vi "Destroy Py Object.vi"(8 "error in (no error)":errorcluster, 10 "Python Object Refnum":T1, 11 "Session Handle in":refnum<data-value>) -> (0 "error out":errorcluster, 3 "Session Handle out":refnum<data-value>)   [LabVIEW 2020, in "G-Embedded-Python-Interpreter-Toolkit.lvlib"]
uses:
  G-Embedded-Python-Interpreter-Toolkit.lvlib
  Python Object Reference.ctl
  Python Object Type.ctl
  bin/gepit.cp310.32.dll
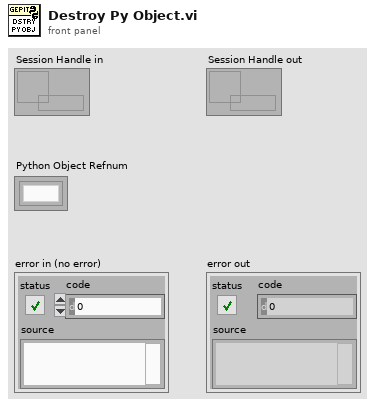
[diagram p1: front panel]
types:
  T1 = typedef "G-Embedded-Python-Interpreter-Toolkit.lvlib/Python Object Reference.ctl" = refnum<k1>
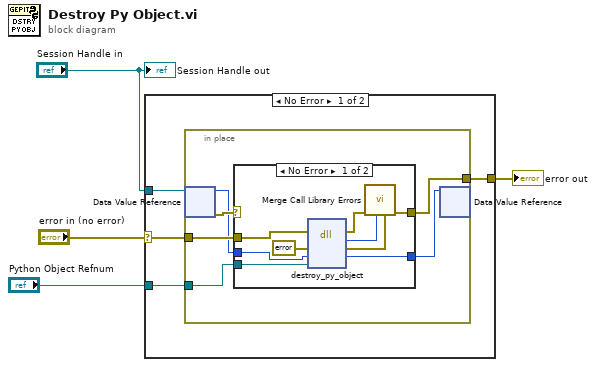
[diagram p0: block diagram]
diagram:
  n1 = case shown="No Error" "error in (no error)" {
    selector: "error in (no error)" -> [w7 w26]
    tunnel: "Session Handle in" -> [w8 _]
    tunnel: [w6 w26] -> w3
    tunnel: "Python Object Refnum" -> [w5 _]
    frame No Error {
      n2 = in-place {
        in-place-border: w7 -> [w13]
        in-place-border: [w10] -> w6
        in-place-border: w5 -> [w9]
        n3 = in-place-dvr #1(w8) -> (w12:u64, w14:errorcluster)
        n4 = case shown="No Error" w14 {
          selector: w14 -> [_ w24]
          tunnel: w13 -> [w19 _]
          tunnel: w12 -> [w18 w25]
          tunnel: [w17 w25] -> w11
          tunnel: [w16 w24] -> w10
          tunnel: w9 -> [w15 _]
          frame No Error {
            n5 = dll-call lib="C:/serenial/libraries/g-embedded-python-interpreter-toolkit/LabVIEW/bin/gepit.cp310.32.dll" fn="destroy_py_object"(error in=w19, "Error"=errorcluster {"status"=FALSE, "code"=0, "source"=""} ("error constant"), "Session"=w18, "Py Object"=w15) -> (error out=w22:errorcluster, "return type"=w21:i32, "Error"=w20:errorcluster, "Session"=w17:u64)  [unwired: 3 in, 1 out]
            n6 = call "Merge Call Library Errors.vi"("Call Library Error"=w20, "Return Value"=w21, "error in"=w22) -> ("error out"=w16:errorcluster)  [unwired: 8 in]
          }
          frame Error {
          }
        }
        n7 = in-place-dvr #1(w11) -> ()  [unwired: 2 out]
      }
    }
    frame Error {
    }
  }
  "error out" <- w3
  "Session Handle out" <- "Session Handle in"
